vi "automatedDraw.vi"() -> ()   [LabVIEW 2018]
uses:
  <vilib>/Analysis/Matrix/Datatypes/RealMatrix.ctl
  <vilib>/Analysis/Matrix/NI_Matrix.lvlib
panel:
  out "drawing":refnum<vi>(3d-picture)
  out "A x B 3":T1=[[1.0, 0.0, 0.0, 0.0], [0.0, 6.123233995736766e-17, 1.0, 0.0], [0.0, -1.0, 6.123233995736766e-17, 0.0], [0.0, 0.0, 0.0, 1.0]] format="%#_2g"
  in  "Enter initials":string
  out "arm picture":refnum<vi>(3d-picture)
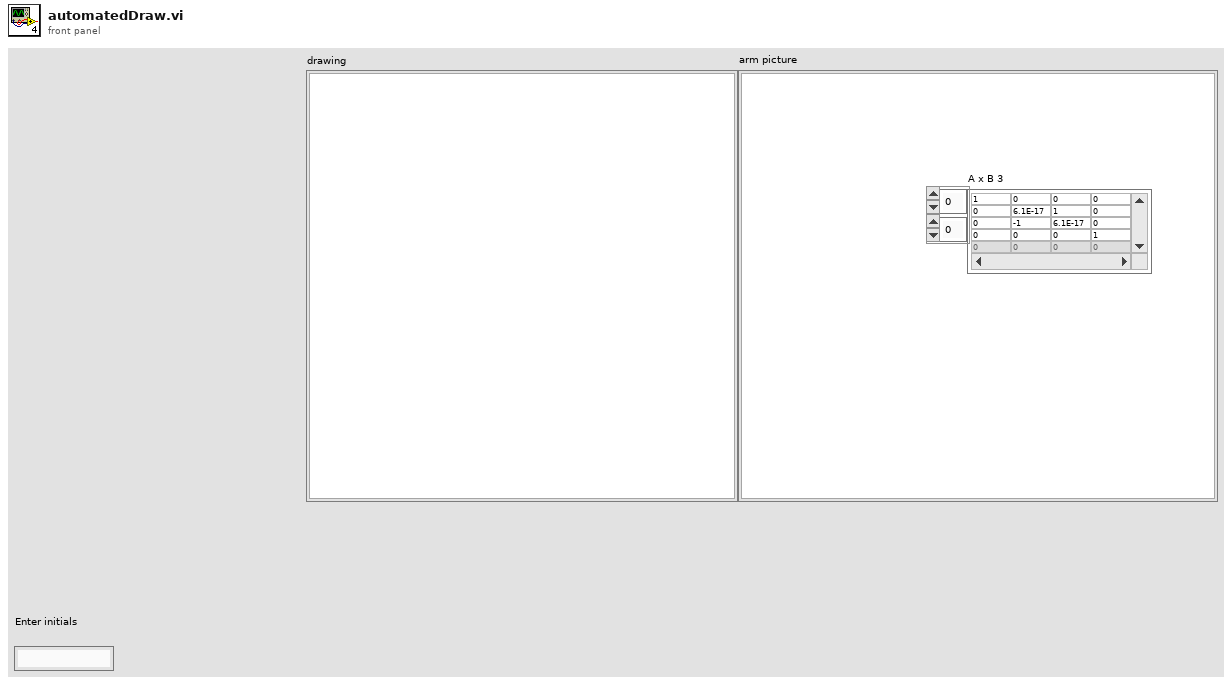
[diagram p1: front panel]
types:
  T1 = typedef "NI_Matrix.lvlib/RealMatrix.ctl" = dbl[][]
  T2 = cluster{"Theta":dbl, "d":dbl, "a":dbl, "alpha (degrees)":dbl}[]
  T3 = cluster{"Theta":dbl, "d":dbl, "a":dbl, "alpha (degrees)":dbl}
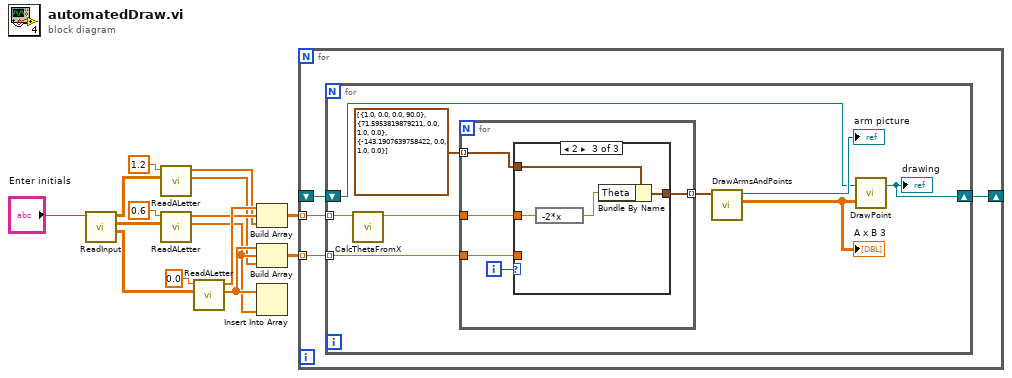
[diagram p0: block diagram]
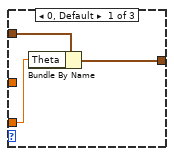
[diagram p2: hidden frame]
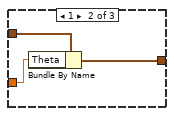
[diagram p3: hidden frame]
diagram:
  n1 = call "ReadInput.vi"("Enter initials"="Enter initials") -> ("all rows 3"=w13:dbl[][], "all rows 2"=w11:dbl[][], "all rows"=w9:dbl[][])  [unwired: 8 in]
  n2 = call "ReadALetter.vi"("all rows 3"=w9, "x"=1.2) -> ("Array 3"=w1:dbl[], "Array 4"=w6:dbl[])  [unwired: 8 in]
  n3 = call "ReadALetter.vi"("all rows 3"=w11, "x"=0.6) -> ("Array 3"=w2:dbl[], "Array 4"=w7:dbl[])  [unwired: 8 in]
  n4 = call "ReadALetter.vi"("all rows 3"=w13, "x"=0.0) -> ("Array 3"=w3:dbl[], "Array 4"=w8:dbl[])  [unwired: 8 in]
  n5 = Build Array(w8, w7, w6) -> (w4:dbl[][])
  n6 = Build Array(w3, w2, w1) -> (w5:dbl[][])
  n7 = Insert Into Array(array=w3, new element=w2) -> ()  [unwired: 1 in, 1 out]
  n8 = for {
    tunnel: w5 -> [w18] mode=indexing
    shift-right: [w19] -> _
    shift-left: _ -> [w16]
    tunnel: w4 -> [w17] mode=indexing
    n9 = for {
      tunnel: w18 -> [w22] mode=indexing
      tunnel: w17 -> [w21] mode=indexing
      shift-right: [w25] -> w19
      shift-left: w16 -> [w20]
      n10 = call "CalcThetaFromX.vi"("X"=w21) -> ("Numeric"=w23:dbl)  [unwired: 10 in]
      n11 = for {
        tunnel: T2 [{"Theta"=1.0, "d"=0.0, "a"=0.0, "alpha (degrees)"=90.0}, {"Theta"=71.5953819879211, "d"=0.0, "a"=1.0, "alpha (degrees)"=0.0}, {"Theta"=-143.1907639758422, "d"=0.0, "a"=1.0, "alpha (degrees)"=0.0}] ("Joints") -> [w33] mode=indexing
        tunnel: [w32] -> w27 mode=indexing
        tunnel: w23 -> [w30]
        tunnel: w22 -> [w29]
        i -> [w31]
        n12 = case shown="2" w31 {
          tunnel: w30 -> [_ w38 w42]
          tunnel: w33 -> [w36 w39 w43]
          tunnel: [w34 w37 w41] -> w32
          tunnel: w29 -> [w35 _ _]
          frame 0, Default {
            n13 = Bundle By Name(cluster=w36, "Theta"=w35) -> (w34:T3)
          }
          frame 1 {
            n14 = Bundle By Name(cluster=w39, "Theta"=w38) -> (w37:T3)
          }
          frame 2 {
            n15 = expression code="-2*x"(w42) -> (w40:dbl)
            n16 = Bundle By Name(cluster=w43, "Theta"=w40) -> (w41:T3)
          }
        }
      }
      n17 = call "DrawArmsAndPoints.vi"("Array"=w27) -> ("A x B"=w26:T1, "SceneObject out"=→"arm picture":refnum<vi>)  [unwired: 9 in]
      "A x B 3" <- w26
      n18 = call "DrawPoint.vi"("Start"=w26, "Stage in"=w20) -> ("Stage out"=w25:refnum<vi>)  [unwired: 1 in]
      "drawing" <- w25
    }
  }
